vi "testPerformZeroCorrection.vi"() -> ()   [LabVIEW 2016]
uses:
  Electrometer/Electrometer.lvclass
  ElectrometerConfiguration/ElectrometerConfiguration.lvclass
panel:
  out "Error Code":i32[](array[numeric])
  out "Error Message":string
  out "error out":errorcluster
  in  "VISA":refnum<visa-resource-name>
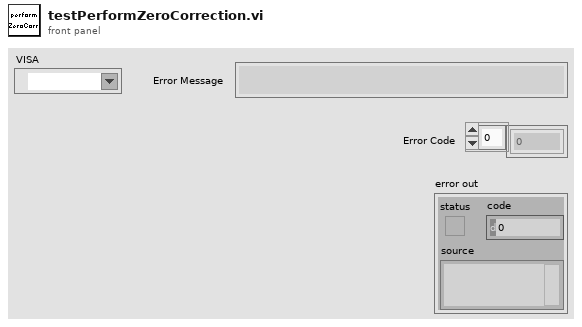
[diagram p1: front panel]
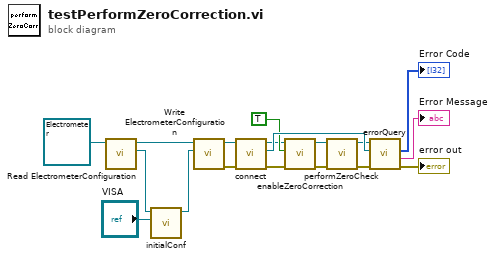
[diagram p0: block diagram]
diagram:
  n1 = call-dynamic "Read ElectrometerConfiguration.vi"("Electrometer in"=refnum<class "Electrometer.lvclass"> refnum ("Electrometer.lvclass")) -> ("ElectrometerConfiguration"=w17:refnum<class "ElectrometerConfiguration.lvclass">, "Electrometer out"=w14:refnum<class "Electrometer.lvclass">)  [unwired: 8 in, 1 out]
  n2 = call "initialConf.vi"("VISA"="VISA", "ElectrometerConfiguration In"=w17) -> ("ElectrometerConfiguration Out"=w15:refnum<class "ElectrometerConfiguration.lvclass">)  [unwired: 9 in]
  n3 = call-dynamic "Write ElectrometerConfiguration.vi"("ElectrometerConfiguration"=w15, "Electrometer in"=w14) -> ("error out"=w13:errorcluster, "Electrometer out"=w12:refnum<class "Electrometer.lvclass">)  [unwired: 8 in]
  n4 = call "connect.vi"("error in (no error)"=w13, "Electrometer in"=w12) -> ("error out"=w5:errorcluster, "VISA resource name"=w11:refnum<visa-resource-name>, "Electrometer out"=w6:refnum<class "Electrometer.lvclass">)  [unwired: 7 in]
  n5 = call "enableZeroCorrection.vi"("error in (no error)"=w5, "Enable Zero Check (T: Enable)"=TRUE, "Electrometer in"=w6) -> ("error out"=w4:errorcluster, "Electrometer out"=w3:refnum<class "Electrometer.lvclass">)  [unwired: 7 in]
  n6 = call "performZeroCheck.vi"("error in (no error)"=w4, "Electrometer in"=w3) -> ("error out"=w1:errorcluster, "Electrometer out"=w2:refnum<class "Electrometer.lvclass">)  [unwired: 8 in]
  n7 = call "errorQuery.vi"("error in (no error)"=w1, "VISA resource name"=w11, "Electrometer in"=w2) -> ("error out"=→"error out":errorcluster, "Error Message"=→"Error Message":string, "Error Code"=→"Error Code":i32[])  [unwired: 5 in, 1 out]
